vi "Query Multi Eval Meas Spectrum Average Limit Check Results.vi"(8 "error in (no error)":errorcluster, 10 "Instance (1)":i32=1, 11 "VISA resource name":refnum<visa-resource-name>) -> (0 "error out":errorcluster, 1 "Out Of Tolerance":i32, 2 "Reliability":i32, 3 "VISA resource name out":refnum<visa-resource-name>, 4 "Results":dbl[](array[numeric]))   [LabVIEW 2020, in "Rohde&Schwarz CMP LR WPAN Measurement.lvlib"]
doc: "Returns the average limit check results. Returns string of 22 single values.\n\nAttribute:\n-\n\nRemote-control command:\nCALCulate:WPAN:MEAS<i>:MEValuation:SPECtrum:AVERage?"
uses:
  <instrlib>/Rohde&Schwarz CMP LR WPAN Measurement/Rohde&Schwarz CMP LR WPAN Measurement.lvlib
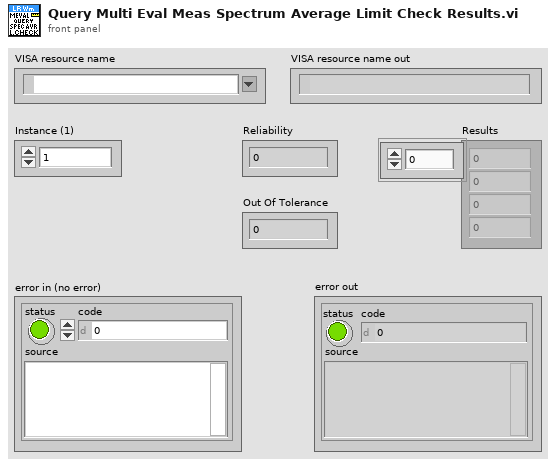
[diagram p1: front panel]
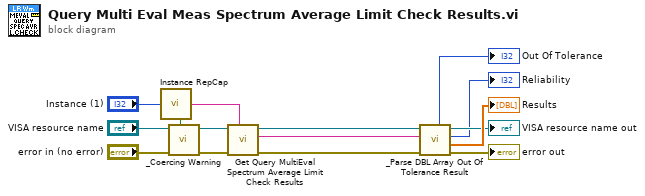
[diagram p0: block diagram]
diagram:
  n1 = call <instrlib>:"Instance RepCap.vi"("Instance In"="Instance (1)") -> ("In Range?"=w15:bool, "RepCap Identifier Out"=w14:string)  [unwired: 1 in]
  n2 = call <instrlib>:"_Coercing Warning.vi"("In Range?"=w15, "error in (no error)"="error in (no error)", "VISA resource name"="VISA resource name") -> ("error out"=w9:errorcluster, "VISA resource name out"=w8:refnum<visa-resource-name>)  [unwired: 7 in]
  n3 = call "Get Query MultiEval Spectrum Average Limit Check Results"("Repeated Capabilities"=w14, "error in (no error)"=w9, "instrument handle"=w8) -> ("error out"=w7:errorcluster, "Query MultiEval Spectrum Average Limit Check Results"=w3:string, "instrument handle out"=w6:refnum<visa-resource-name>)  [unwired: 6 in]
  n4 = call <instrlib>:"_Parse DBL Array Out Of Tolerance Result.vi"("error in (no error)"=w7, "Input String"=w3, "VISA resource name"=w6) -> ("error out"=→"error out":errorcluster, "Results"=→"Results":dbl[], "Reliability"=→"Reliability":i32, "VISA resource name out"=→"VISA resource name out":refnum<visa-resource-name>, "Out Of Tolerance"=→"Out Of Tolerance":i32)  [unwired: 4 in]
